vi "control panel globals.vi"() -> ()   [LabVIEW 2017]
uses:
  typedefs/queue cluster.ctl
  typedefs/reading queue.ctl
  typedefs/reading.ctl
  typedefs/readingType.ctl
  typedefs/magnetomter reading set.ctl
  typedefs/magnetic field fit.ctl
panel:
  in  "g (m/s^2)":dbl=9.802
  in  "bob mass":dbl=0.55
  in  "magnet height":dbl=0.039
  out "screenshot queue":refnum<queue>
  in  "main vi ref":refnum<vi>
  out "ellipse fit":T1
  out "crossing stats":T2
  out "pulse statistics":T3 {"timing error" format="%#.3p"}
  out "initialized":bool
  out "disk queues":T4
  out "display queues":T4
  out "stop":bool
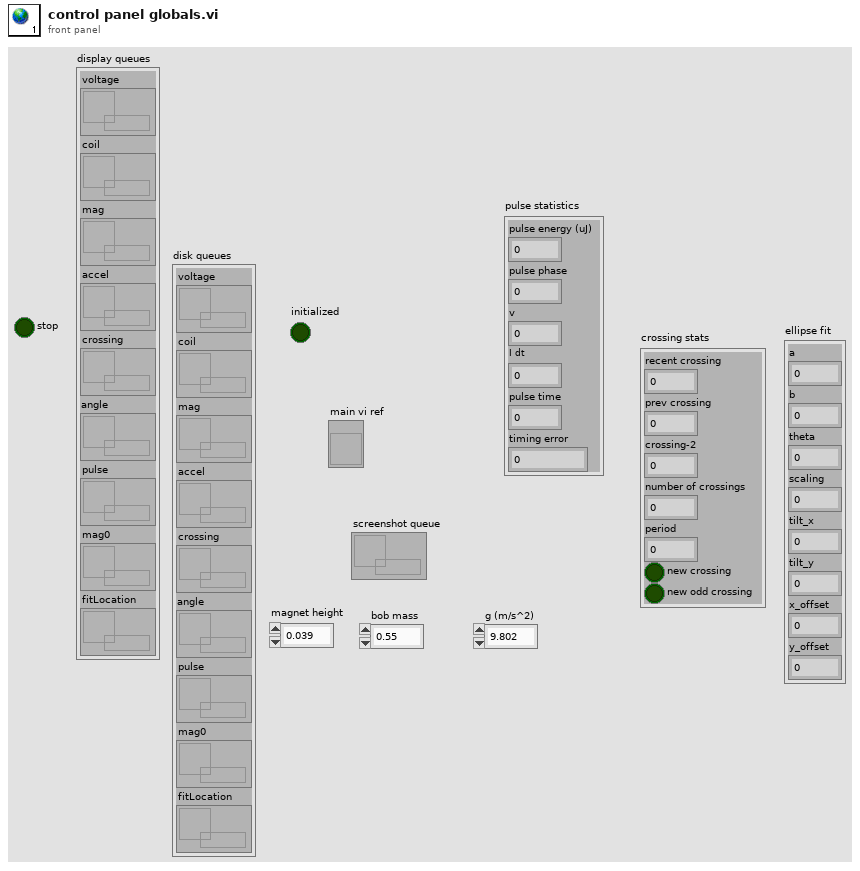
[diagram p1: front panel]
types:
  T1 = typedef "magnetic field fit.ctl" = cluster{"a":dbl, "b":dbl, "theta":dbl, "scaling":dbl, "tilt_x":dbl, "tilt_y":dbl, "bx_offset":dbl, "by_offset":dbl, "bz_offset":dbl, "x_offset":dbl, "y_offset":dbl}
  T2 = cluster{"recent crossing":dbl, "prev crossing":dbl, "crossing-2":dbl, "number of crossings":i32, "period":dbl, "new crossing":bool, "new odd crossing":bool}
  T3 = cluster{"pulse energy (uJ)":sgl, "pulse phase":dbl, "v":dbl, "I dt":dbl, "pulse time":dbl, "timing error":dbl}
  T4 = typedef "queue cluster.ctl" = cluster{"voltage":T5, "coil":T5, "mag":refnum<queue>, "accel":T5, "crossing":T5, "angle":T5, "pulse":T5, "mag0":T5, "fitLocation":T5}
  T5 = typedef "reading queue.ctl" = refnum<queue>
diagram:
